vi "LWXPS_Equals.vi"(3 "LabVIEW error IN":errorcluster, 4 "obj":refnum<k24>, 5 "XPS Reference IN":refnum<k24>) -> (0 "LabVIEW error OUT":errorcluster, 1 "Equals":bool, 2 "XPS Reference OUT":refnum<k24>)   [LabVIEW 2014]
uses:
  D:/XPSQ8_LabView_Library/Development/Source/Dll/Newport.XPS.CommandInterface.dll
  Dll/Newport.XPS.CommandInterface.dll
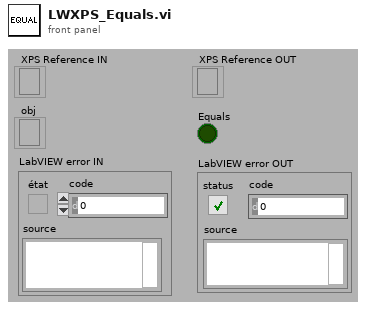
[diagram p1: front panel]
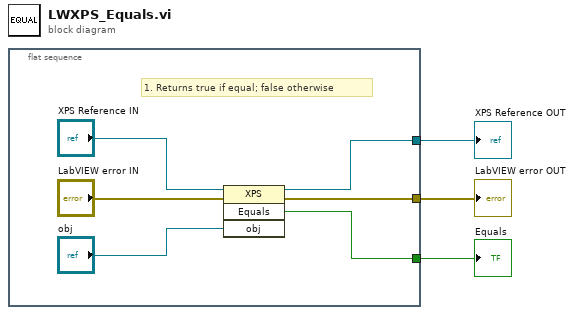
[diagram p0: block diagram]
diagram:
  n1 = flat-sequence {
    tunnel: [w6] -> w3
    tunnel: [w9] -> w2
    tunnel: [w4] -> w1
    frame #0 {
      # "1. Returns true if equal; false otherwise"
      n2 = invoke class="XPS" method="Equals"(reference="XPS Reference IN", error in="LabVIEW error IN", "obj"="obj") -> (reference out=w6:refnum<k24>, error out=w9:errorcluster, "Equals"=w4:bool)  [unwired: 1 in, 1 out]
    }
  }
  "XPS Reference OUT" <- w3
  "LabVIEW error OUT" <- w2
  "Equals" <- w1
